vi "Sphere Fit.vi"() -> ()   [LabVIEW 2023]
doc: "Determines the best spherical fit on a cloud of points in 3D. You can fix the number of points and the midpoint and radius of the sphere in 3D. A random factor can be applied to the generated points (a factor of 0 will generate points exactly on the surface of the sphere). The generated cloud of points is fitted and the result is displayed in the 3D Picture."
uses:
  <vilib>/picture/3D Picture Control/Object/Create Object (drawable).vi
  <vilib>/picture/3D Picture Control/Object/Create Object (drawable with reference).vi
  <vilib>/picture/3D Picture Control/Object/Add Object (no reference).vi
  <vilib>/gmath/NI_Gmath.lvlib
  <vilib>/picture/3D Picture Control/NI_3D Picture Control.lvlib
panel:
  in  "Transparency":sgl(slide)=0.4 scale=0.0..1.0
  in  "Stop":bool
  out "3D Picture":refnum<vi>(3d-picture)
  in  "Random Factor":dbl=0.2
  out "Calculated Radius":dbl
  out "Calculated [x0, y0, z0]":dbl[](array[numeric]) format="%#.6g"
  in  "Radius":dbl=1.0
  in  "Z":dbl
  in  "Y":dbl
  in  "X":dbl
  in  "Number of points":i32=100
  # "Overview: Demonstrates how to fit spherical data with the Fitting on a Sphere VI and display the fit data in a 3D Picture.\nRequirements: LabVIEW Full Development System\nInstructions: \n1. Set the X,Y,Z, and Radius of the sphere. Also set the Random Factor to to generate points outside the sphere.\n2. Run the VI and verify the resulting sphere and its calculated radius and center. Manipulate the view of the 3D Picture by dragging, shift-dragging, or control-dragging in the image area.\n3. Click Stop to stop the VI."
  # "Fitting on a Sphere"
  # "Fitting points to sphere"
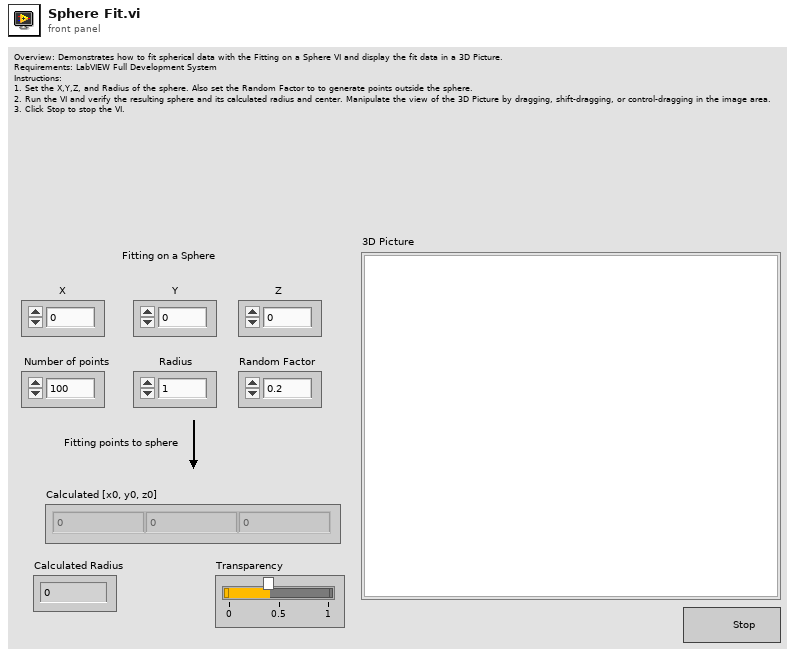
[diagram p1: front panel]
types:
  T1 = enum16{"Inherit Value", "Points", "Wireframe", "Polygons"}
  T2 = enum16{"Normal Bin", "Opaque Bin", "Transparent Bin"}
  T3 = enum16{"Points", "Lines", "Line Strip", "Line Loop", "Triangles", "Triangle Strip", "Triangle Fan", "Quads", "Quad Strip", "Polygon"}
  T4 = cluster{"x0, y0, z0[0]":dbl, "x0, y0, z0[1]":dbl, "x0, y0, z0[2]":dbl}
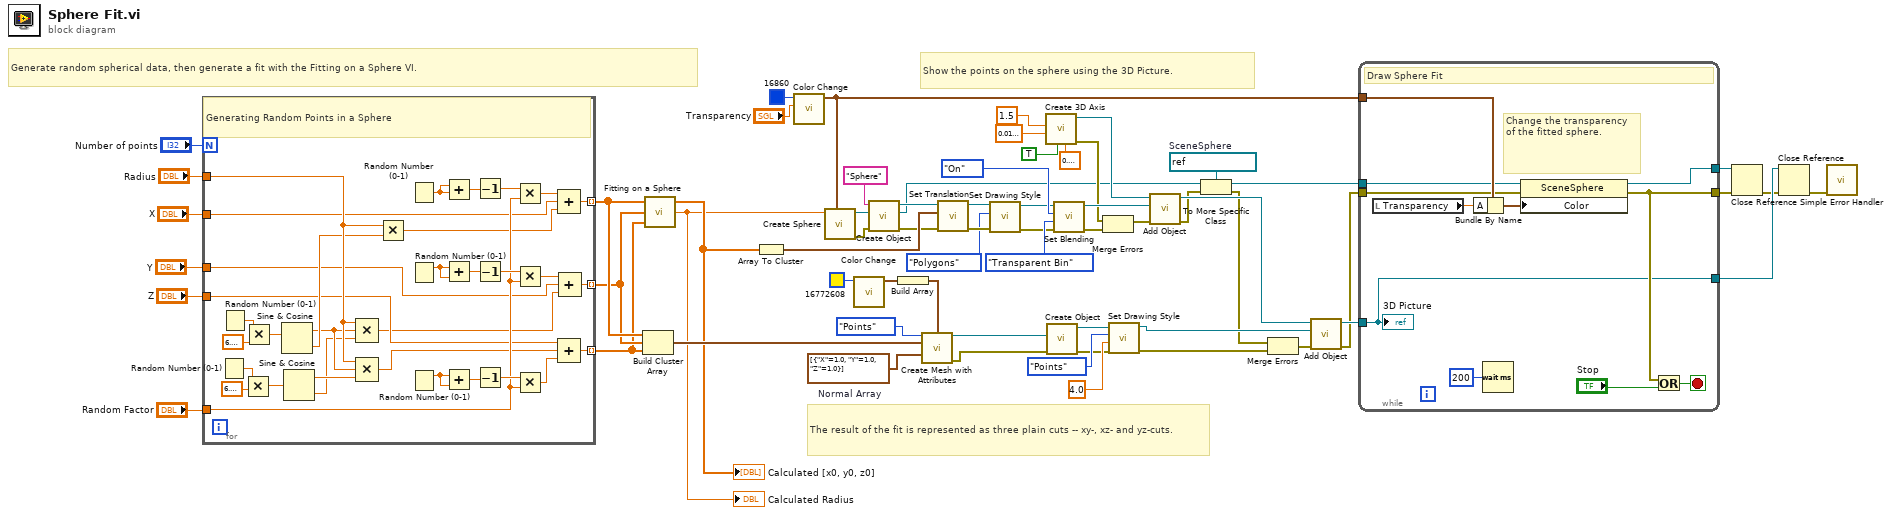
[diagram p0: block diagram]
diagram:
  w12 = refnum<vi> refnum  # SceneSphere
  w9 = cluster{"X":sgl, "Y":sgl, "Z":sgl}[] [{"X"=1.0, "Y"=1.0, "Z"=1.0}]  # Normal Array
  # "The result of the fit is represented as three plain cuts -- xy-, xz- and yz-cuts."
  # "Generate random spherical data, then generate a fit with the Fitting on a Sphere VI."
  # "Show the points on the sphere using the 3D Picture."
  n1 = for {
    N: "Number of points" -> [_]
    tunnel: "Radius" -> [w79]
    tunnel: "X" -> [w68]
    tunnel: "Y" -> [w74]
    tunnel: "Z" -> [w75]
    tunnel: [w67] -> w37 mode=indexing
    tunnel: [w80] -> w36 mode=indexing
    tunnel: [w91] -> w35 mode=indexing
    tunnel: "Random Factor" -> [w76]
    # "Generating Random Points in a Sphere"
    n2 = Random Number (0-1)() -> (number: 0 to 1=w94:dbl)
    n3 = Random Number (0-1)() -> (number: 0 to 1=w97:dbl)
    n4 = Multiply(x=w94, y=6.283185307179586) -> (x*y=w93:dbl)
    n5 = Multiply(x=w97, y=6.283185307179586) -> (x*y=w77:dbl)
    n6 = Sine & Cosine(0:w77) -> (1:w71:dbl, 2:w78:dbl)
    n7 = Sine & Cosine(0:w93) -> (1:w72:dbl, 2:w70:dbl)
    n8 = Compound Arithmetic op=MULTIPLY(w79, w71, w70) -> (w73:dbl)
    n9 = Compound Arithmetic op=MULTIPLY(w79, w71, w72) -> (w65:dbl)
    n10 = Multiply(x=w79, y=w78) -> (x*y=w69:dbl)
    n11 = Random Number (0-1)() -> (number: 0 to 1=w90:dbl)
    n12 = Random Number (0-1)() -> (number: 0 to 1=w83:dbl)
    n13 = Random Number (0-1)() -> (number: 0 to 1=w87:dbl)
    n14 = Add(x=w90, y=w90) -> (x+y=w89:dbl)
    n15 = Add(x=w83, y=w83) -> (x+y=w84:dbl)
    n16 = Add(x=w87, y=w87) -> (x+y=w86:dbl)
    n17 = Decrement(x=w89) -> (x-1=w88:dbl)
    n18 = Decrement(x=w84) -> (x-1=w82:dbl)
    n19 = Decrement(x=w86) -> (x-1=w85:dbl)
    n20 = Multiply(x=w88, y=w76) -> (x*y=w92:dbl)
    n21 = Multiply(x=w82, y=w76) -> (x*y=w81:dbl)
    n22 = Multiply(x=w85, y=w76) -> (x*y=w66:dbl)
    n23 = Compound Arithmetic op=ADD(w92, w68, w69) -> (w67:dbl)
    n24 = Compound Arithmetic op=ADD(w75, w65, w66) -> (w91:dbl)
    n25 = Compound Arithmetic op=ADD(w81, w74, w73) -> (w80:dbl)
  }
  n26 = Build Cluster Array(w37, w36, w35) -> (w57:cluster{dbl, dbl, dbl}[])
  n27 = call <vilib>:"Fitting on a Sphere.vi"("Z"=w35, "Y"=w36, "X"=w37) -> ("r"=w8:dbl, "x0, y0, z0"=w34:dbl[])  [unwired: 1 out]
  "Calculated [x0, y0, z0]" <- w34
  "Calculated Radius" <- w8
  n28 = Array To Cluster(array=w34) -> (cluster=w42:T4)
  n29 = call <vilib>:"Color Change.vi"("Alpha"="Transparency", "Color"=u32 16860) -> ("RGBA"=w18:cluster{"R":sgl, "G":sgl, "B":sgl, "A":sgl})  [unwired: 9 in]
  n30 = call <vilib>:"Create Sphere.vi"("Color"=w18, "Radius"=w8) -> ("error out"=w28:errorcluster, "New Sphere Refnum"=w23:refnum<vi>)  [unwired: 8 in]
  n31 = call <vilib>:"Color Change.vi"("Color"=u32 16772608) -> ("RGBA"=w44:cluster{"R":sgl, "G":sgl, "B":sgl, "A":sgl})  [unwired: 10 in]
  n32 = call-poly <vilib>:"Create Object.vi"("error in (no error)"=w28, "Geometry or text"=w23, "Name"="Sphere") -> ("error out"=w29:errorcluster, "Drawable refnum"=w11:refnum<vi>, "Scene:New Object"=w43:refnum<vi>)  [unwired: 6 in]
  n33 = Build Array(w44) -> (w45:cluster{"R":sgl, "G":sgl, "B":sgl, "A":sgl}[])
  n34 = call <vilib>:"Create Mesh with Attributes.vi"("Draw Mode"=T3."Points", "Color Array"=w45, "Vertex Array"=w57, "Normal Array"=w9) -> ("New Mesh Refnum"=w56:refnum<vi>, "error out"=w33:errorcluster)  [unwired: 10 in]
  n35 = call <vilib>:"Set Translation.vi"("error in (no error)"=w29, "Translation"=w42, "Scene Object"=w43) -> ("error out"=w17:errorcluster, "Translated Object"=w16:refnum<vi>)  [unwired: 7 in]
  n36 = call <vilib>:"Set Drawing Style.vi"("error in (no error)"=w17, "Mode"=T1."Polygons", "Scene Object In"=w16) -> ("error out"=w14:errorcluster, "Scene Object Out"=w15:refnum<vi>)  [unwired: 7 in]
  n37 = call <vilib>:"Create 3D Axis.vi"("Character Size"=sgl 0.2, "Axis label?"=TRUE, "Radius"=sgl 0.02, "Length"=sgl 1.5) -> ("error out"=w26:errorcluster, "New Object Refnum"=w53:refnum<vi>)  [unwired: 6 in]
  n38 = call-poly <vilib>:"Create Object.vi"("error in (no error)"=w33, "Geometry"=w56) -> ("error out"=w32:errorcluster, "Scene:New Object"=w55:refnum<vi>)  [unwired: 8 in]
  n39 = call <vilib>:"Set Blending.vi"("error in (no error)"=w14, "Bin"=T2."Transparent Bin", "Mode"=enum16{"Inherit Value", "Off", "On"}."On", "Scene Object In"=w15) -> ("error out"=w27:errorcluster, "Scene Object Out"=w50:refnum<vi>)  [unwired: 6 in]
  n40 = Merge Errors(w26, w27) -> (w25:errorcluster)
  n41 = call <vilib>:"Set Drawing Style.vi"("error in (no error)"=w32, "Size"=4.0, "Mode"=T1."Points", "Scene Object In"=w55) -> ("error out"=w31:errorcluster, "Scene Object Out"=w47:refnum<vi>)  [unwired: 6 in]
  n42 = call-poly <vilib>:"Add Object.vi"("error in (no error)"=w25, "New Object In"=w50, "Scene Object In"=w53) -> ("error out"=w7:errorcluster, "Scene Object Out"=w52:refnum<vi>)  [unwired: 7 in]
  n43 = To More Specific Class(target class=w12, reference=w11, error in=w7) -> (specific class reference=w10:refnum<vi>, error out=w6:errorcluster)
  n44 = Merge Errors(w6, w31) -> (w30:errorcluster)
  n45 = call-poly <vilib>:"Add Object.vi"("error in (no error)"=w30, "New Object In"=w47, "Scene Object In"=w52) -> ("error out"=w19:errorcluster, "Scene Object Out"=w24:refnum<vi>)  [unwired: 7 in]
  n46 = while {
    tunnel: w24 -> [w98]
    tunnel: w19 -> [w100]
    tunnel: [w102] -> w3
    tunnel: w18 -> [w105]
    tunnel: w10 -> [w101]
    tunnel: [w99] -> w5
    tunnel: [w98] -> w4
    stop <- w108 stop-if-true
    # "Change the transparency of the fitted sphere."
    # "Draw Sphere Fit"
    n47 = local read "Transparency"() -> (w104:sgl)
    n48 = Bundle By Name(cluster=w105, "A"=w104) -> (w103:cluster{"R":sgl, "G":sgl, "B":sgl, "A":sgl})
    n49 = Wait (ms)(milliseconds to wait=u32 200) -> ()  [unwired: 1 out]
    n50 = property class="SceneSphere"(reference=w101, error in=w100, "Color"=w103) -> (reference out=w99:refnum<vi>, error out=w102:errorcluster)
    n51 = Or(x=w102, y="Stop") -> (x .or. y?=w108:bool)
    "3D Picture" <- w98
  }
  n52 = Close Reference(reference=w5, error in (no error)=w3) -> (error out=w2:errorcluster)
  n53 = Close Reference(reference=w4, error in (no error)=w2) -> (error out=w1:errorcluster)
  n54 = call <vilib>:"Simple Error Handler.vi"("error in (no error)"=w1) -> ()  [unwired: 4 in, 5 out]
